vi "Calculate Polynomial.vi"(1 "Coefficients":sgl[](array[numeric]), 2 "Value":sgl) -> (0 "Result":sgl)   [LabVIEW 2021]
panel:
  # "x^2+2x+3"
  # "x=4"
  # "y=27"
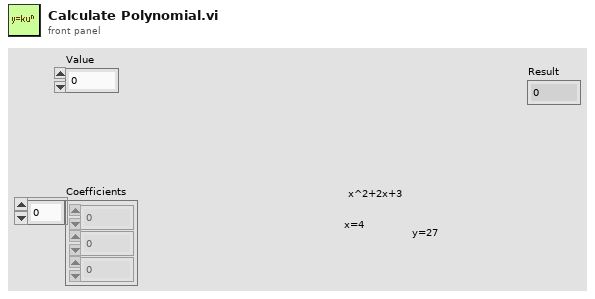
[diagram p1: front panel]
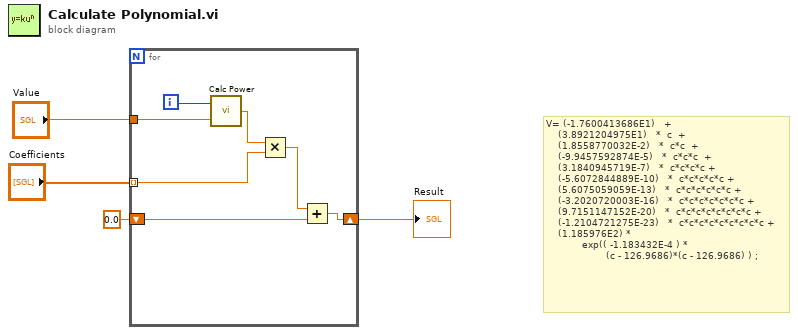
[diagram p0: block diagram]
diagram:
  # "V= (-1.7600413686E1)   +\n    (3.8921204975E1)   *  c  +\n    (1.8558770032E-2)   *  c*c  +\n    (-9.9457592874E-5)   *  c*c*c  +\n    (3.1840945719E-7)   *  c*c*c*c +\n    (-5.6072844889E-10)   *  c*c*c*c*c +\n    (5.6075059059E-13)   *  c*c*c*c*c*c +\n    (-3.2020720003E-16)   *  c*c*c*c*c*c*c +\n    (9.7151147152E-20)   *  c*c*c*c*c*c*c*c +\n    (-1.2104721275E-23)   *  c*c*c*c*c*c*c*c*c +\n    (1.185976E2) * \n            exp(( -1.183432E-4 ) * \n                    (c - 126.9686)*(c - 126.9686) ) ;"
  n1 = for {
    tunnel: "Coefficients" -> [w8] mode=indexing
    shift-right: [w10] -> w1
    shift-left: sgl 0.0 -> [w5]
    tunnel: "Value" -> [w9]
    i -> [w11]
    n2 = call "Calc Power.vi"("Value"=w9, "Power"=w11) -> ("Result"=w7:sgl)
    n3 = Multiply(x=w7, y=w8) -> (x*y=w6:sgl)
    n4 = Add(x=w6, y=w5) -> (x+y=w10:sgl)
  }
  "Result" <- w1
